vi "ScaleTorque.vi"(6 "Scale Dir":T1=enum."Full scale -> Model scale", 8 "Scale factor":dbl, 11 "Torque (In)":dbl) -> (3 "Torque (Out)":dbl)   [LabVIEW 2018]
uses:
  Clusters/ScalingEnum.ctl
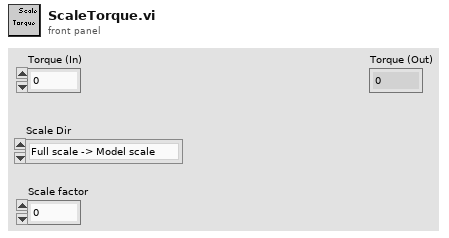
[diagram p1: front panel]
types:
  T1 = typedef "ScalingEnum.ctl" = enum16{"Model scale -> Full scale", "Full scale -> Model scale"}
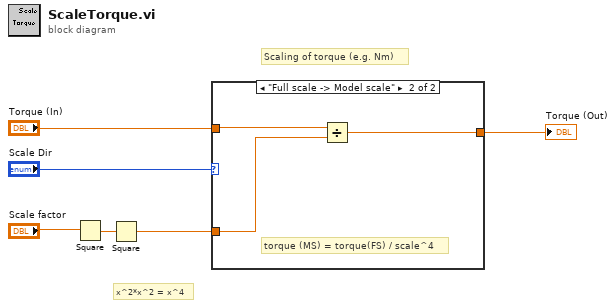
[diagram p0: block diagram]
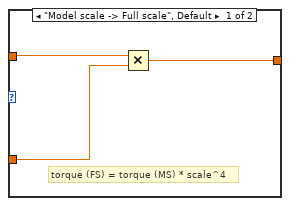
[diagram p2: hidden frame]
diagram:
  # "x^2*x^2 = x^4"
  # "Scaling of torque (e.g. Nm)"
  n1 = Square(x="Scale factor") -> (x^2=w2:dbl)
  n2 = Square(x=w2) -> (x^2=w1:dbl)
  n3 = case shown="\"Full scale -> Model scale\"" "Scale Dir" {
    tunnel: "Torque (In)" -> [w9 w12]
    tunnel: w1 -> [w8 w11]
    tunnel: [w7 w10] -> w4
    frame "Model scale -> Full scale", Default {
      # "torque (FS) = torque (MS) * scale^4"
      n4 = Multiply(x=w9, y=w8) -> (x*y=w7:dbl)
    }
    frame "Full scale -> Model scale" {
      # "torque (MS) = torque(FS) / scale^4"
      n5 = Divide(x=w12, y=w11) -> (x/y=w10:dbl)
    }
  }
  "Torque (Out)" <- w4
